vi "CV_BuildPoints.vi"(0 "Number Of Loops":i32, 1 "Jump At Start":bool, 9 "V Positions":dbl[](array[numeric])=[0.0, 0.0, 0.0], 11 "V Velocities":dbl[](array[numeric])=[0.0, 0.0, 0.0]) -> (10 "V Positions":dbl[](array[numeric]), 12 "V Move":bool[](array[boolean]), 13 "V Velocities":dbl[](array[numeric]), 15 "JumpV":bool[](array[boolean]))   [LabVIEW 2023]
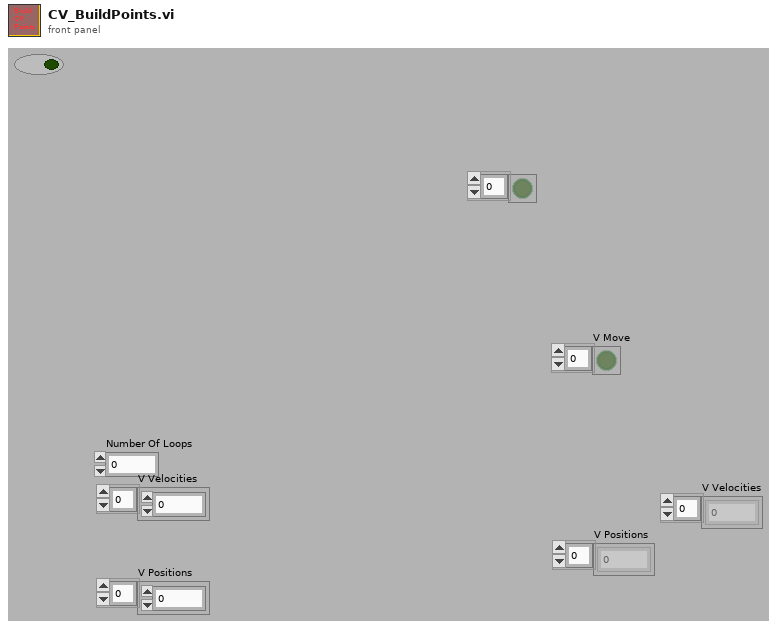
[diagram p1: front panel]
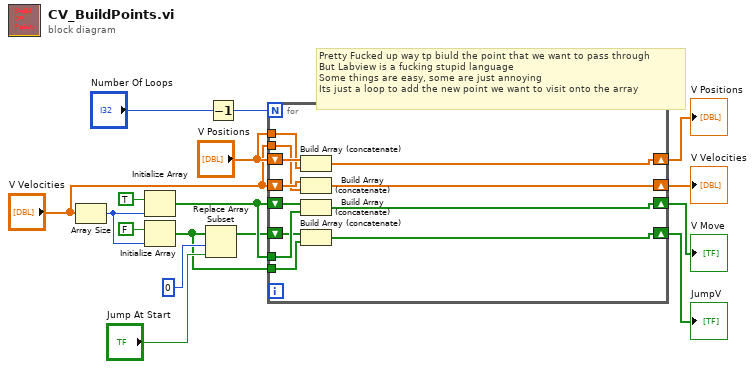
[diagram p0: block diagram]
diagram:
  # "Pretty Fucked up way tp biuld the point that we want to pass through\nBut Labview is a fucking stupid language\nSome things are easy, some are just annoying\nIts just a loop to add the new point we want to visit onto the array"
  n1 = Array Size(array="V Velocities") -> (size(s)=w6:i32)
  n2 = Initialize Array(TRUE, w6) -> (w8:bool[])
  n3 = Initialize Array(FALSE, w6) -> (w2:bool[])
  n4 = Replace Array Subset(array=w2, new element="Jump At Start", index=0) -> (w1:bool[])
  n5 = Decrement(x="Number Of Loops") -> (x-1=w16:i32)
  n6 = for {
    N: w16 -> [_]
    shift-right: [w27] -> w14
    shift-left: "V Positions" -> [w28]
    shift-right: [w26] -> w12
    shift-left: "V Velocities" -> [w25]
    tunnel: "V Positions" -> [w20]
    tunnel: "V Velocities" -> [w24]
    tunnel: w8 -> [w22]
    shift-right: [w21] -> w11
    shift-left: w8 -> [w23]
    shift-right: [w17] -> w5
    shift-left: w1 -> [w19]
    tunnel: w2 -> [w18]
    n7 = Build Array (concatenate)(w28, w20) -> (w27:dbl[])
    n8 = Build Array (concatenate)(w25, w24) -> (w26:dbl[])
    n9 = Build Array (concatenate)(w23, w22) -> (w21:bool[])
    n10 = Build Array (concatenate)(w19, w18) -> (w17:bool[])
  }
  "V Positions" <- w14
  "V Velocities" <- w12
  "V Move" <- w11
  "JumpV" <- w5
